vi "Fetch Multi Eval Meas IEM Margin RB Index Results.vi"(8 "error in (no error)":errorcluster, 9 "Result Type (Current)":i32(ring) items=["Current"=0, "Extreme"=2], 10 "Instance (1)":T2=1, 11 "VISA resource name":refnum<visa-resource-name>) -> (0 "error out":errorcluster, 1 "Margin RB Index Results":T1 {"Out Of Tolerance" format="%^.3e"}, 2 "Reliability":i32, 3 "VISA resource name out":refnum<visa-resource-name>)   [LabVIEW 2015, in "Rohde&Schwarz CMXP NR FR2 Measurement.lvlib"]
doc: "Returns the multi eval measurement IEM limit line margin RB index results.\n\nAttributes:\nRSCMXPNRFR2M_ATTR_FETCH_MULTI_EVAL_MEASUREMENT_IEM_MARGIN_RB_INDEX_CURRENT_RESULTS\nRSCMXPNRFR2M_ATTR_FETCH_MULTI_EVAL_MEASUREMENT_IEM_MARGIN_RB_INDEX_EXTREME_RESULTS\n\nRemote-control commands:\nFETCh:NRMMw:MEAS<i>:MEValuation:IEMission:MARGin:CURRent:RBINdex?\nFETCh:NRMMw:MEAS<i>:MEValuation:IEMission:MARGin:EXTReme:RBINdex?"
uses:
  <instrlib>/Rohde&Schwarz CMXP NR FR2 Measurement/Rohde&Schwarz CMXP NR FR2 Measurement.lvlib
  <instrlib>/Rohde&Schwarz CMXP NR FR2 Measurement/Private/_Instance.ctl
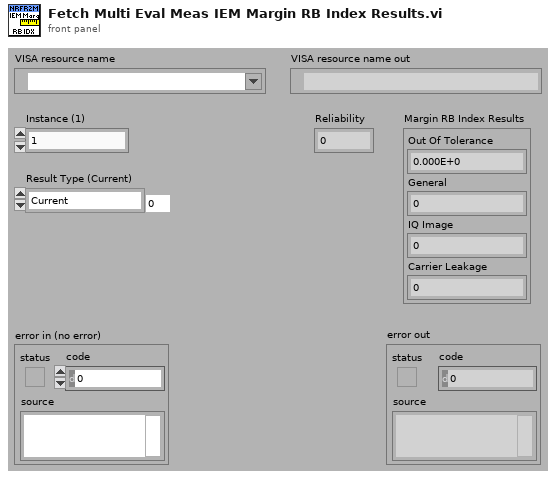
[diagram p1: front panel]
types:
  T1 = cluster{"Out Of Tolerance":dbl, "General":i32, "IQ Image":i32, "Carrier Leakage":i32}
  T2 = typedef "Rohde&Schwarz CMXP NR FR2 Measurement.lvlib/_Instance.ctl" = i32
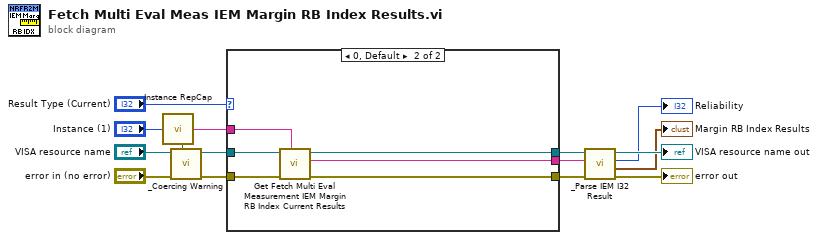
[diagram p0: block diagram]
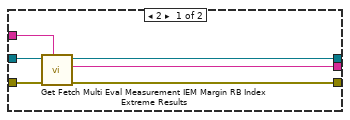
[diagram p2: hidden frame]
diagram:
  n1 = call <instrlib>:"Instance RepCap.vi"("Instance In"="Instance (1)") -> ("In Range?"=w3:bool, "RepCap Identifier Out"=w14:string)  [unwired: 1 in]
  n2 = call <instrlib>:"_Coercing Warning.vi"("In Range?"=w3, "error in (no error)"="error in (no error)", "VISA resource name"="VISA resource name") -> ("error out"=w4:errorcluster, "VISA resource name out"=w5:refnum<visa-resource-name>)  [unwired: 7 in]
  n3 = case shown="0, Default" "Result Type (Current)" {
    tunnel: w4 -> [w21 w27]
    tunnel: w5 -> [w20 w26]
    tunnel: [w19 w25] -> w13
    tunnel: [w18 w24] -> w12
    tunnel: w14 -> [w16 w23]
    tunnel: [w17 w22] -> w8
    frame 2 {
      n4 = call "Get Fetch Multi Eval Measurement IEM Margin RB Index Extreme Results"("Repeated Capabilities"=w16, "error in (no error)"=w21, "instrument handle"=w20) -> ("error out"=w19:errorcluster, "Fetch Multi Eval Measurement IEM Margin RB Index Extreme Results"=w17:string, "instrument handle out"=w18:refnum<visa-resource-name>)  [unwired: 6 in]
    }
    frame 0, Default {
      n5 = call "Get Fetch Multi Eval Measurement IEM Margin RB Index Current Results"("Repeated Capabilities"=w23, "error in (no error)"=w27, "instrument handle"=w26) -> ("error out"=w25:errorcluster, "Fetch Multi Eval Measurement IEM Margin RB Index Current Results"=w22:string, "instrument handle out"=w24:refnum<visa-resource-name>)  [unwired: 6 in]
    }
  }
  n6 = call <instrlib>:"_Parse IEM I32 Result.vi"("error in (no error)"=w13, "Input String"=w8, "VISA resource name"=w12) -> ("error out"=→"error out":errorcluster, "Results"=→"Margin RB Index Results":T1, "Reliability"=→"Reliability":i32, "VISA resource name out"=→"VISA resource name out":refnum<visa-resource-name>)  [unwired: 5 in]
